vi "Create Database.vi"(0 "InfluxDB in":refnum<class "InfluxDB Client.lvclass">, 5 "Database name":string, 11 "error in (no error)":errorcluster) -> (4 "InfluxDB out":refnum<class "InfluxDB Client.lvclass">, 15 "error out":errorcluster)   [LabVIEW 2015, in "InfluxDB Client.lvclass"]
doc: "Creates a database."
uses:
  InfluxDB Client.lvclass
  InfluxDB Client.lvclass/InfluxDB Client.ctl
  <vilib>/httpClient/POSTBuffer.vi
  <vilib>/httpClient/LabVIEWHTTPClient.lvlib
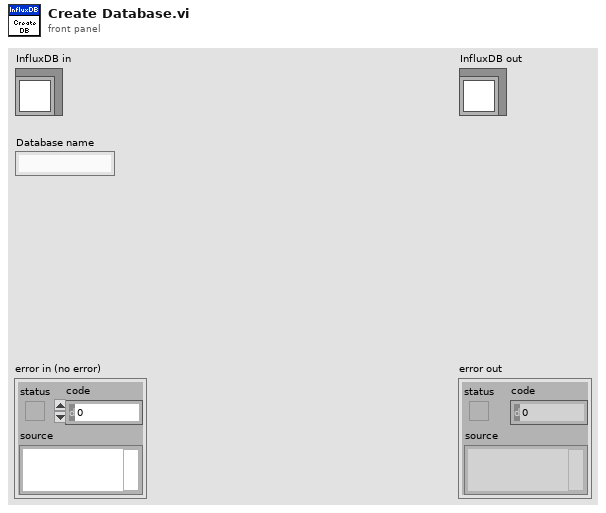
[diagram p1: front panel]
types:
  T1 = typedef "LabVIEWHTTPClient.lvlib/ClientHandle.ctl" = refnum<k1>
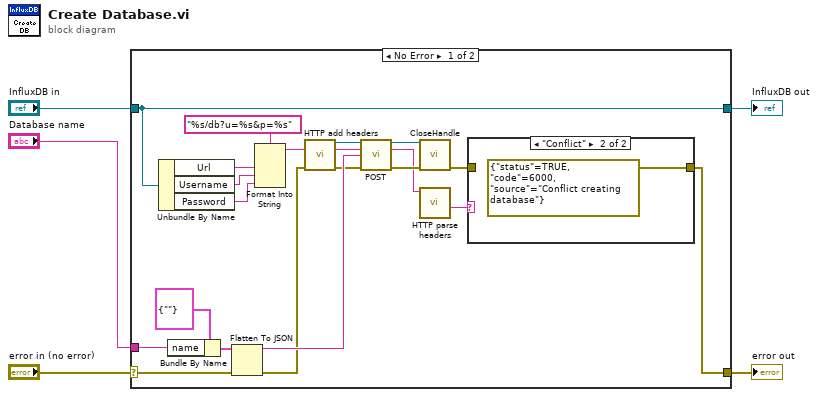
[diagram p0: block diagram]
diagram:
  n1 = case shown="No Error" "error in (no error)" {
    selector: "error in (no error)" -> [w8 w29]
    tunnel: [w10 w29] -> w4
    tunnel: [w25 w28] -> w2
    tunnel: "InfluxDB in" -> [w25 w28]
    tunnel: "Database name" -> [w18 _]
    frame No Error {
      n2 = Unbundle By Name(w25) -> ("Url"=w23:string, "Username"=w22:string, "Password"=w21:string)
      n3 = Bundle By Name(cluster=cluster{"name":string} {"name"=""} ("anything"), "name"=w18) -> (w20:cluster{"name":string})
      n4 = Flatten To JSON(anything=w20, error in (no error)=w8) -> (JSON string=w14:string, 11:w7:errorcluster)  [unwired: 1 in]
      n5 = Format Into String(format string="%s/db?u=%s&p=%s" ("url"), w23, w22, w21) -> (resulting string=w15:string)  [unwired: 2 in, 1 out]
      n6 = call "HTTP add headers.vi"("error in (no error)"=w7) -> ("client handle out"=w9:T1, "error out"=w6:errorcluster)  [unwired: 13 in]
      n7 = call-poly <vilib>:"POST.vi"("client handle"=w9, "url"=w15, "buffer"=w14, "error in (no error)"=w6) -> ("client handle out"=w17:T1, "headers"=w13:string, "error out"=w16:errorcluster)  [unwired: 8 in, 1 out]
      n8 = call <vilib>:"CloseHandle.vi"("client handle"=w17, "error in (no error)"=w16) -> ("error out"=w11:errorcluster)  [unwired: 13 in]
      n9 = call "HTTP parse headers.vi"("HTTP headers"=w13) -> ("Status"=w12:string)  [unwired: 8 in, 2 out]
      n10 = case shown="\"Conflict\"" w12 {
        tunnel: w11 -> [w26 _]
        tunnel: [w26 errorcluster {"status"=TRUE, "code"=6000, "source"="Conflict creating database"} ("error constant")] -> w10
        frame Default {
        }
        frame "Conflict" {
        }
      }
    }
    frame Error {
    }
  }
  "error out" <- w4
  "InfluxDB out" <- w2
